vi "video.create_begin.vi"(8 "error in":errorcluster, 10 "name":string, 11 "Client in":refnum<class "Client.lvclass">) -> (0 "error out":errorcluster, 2 "VideoCreateStaging":refnum<class "VideoCreateStaging.lvclass">, 3 "Client out":refnum<class "Client.lvclass">)   [LabVIEW 2020, in "Client.lvclass"]
doc: "Creates a new empty video (metadata shell) with a name and optional description in Nominal and returns a handle to it."
uses:
  Client.lvclass
  Client.lvclass/Client.ctl
  client.lvlib
  VideoCreateStaging/VideoCreateStaging.lvclass
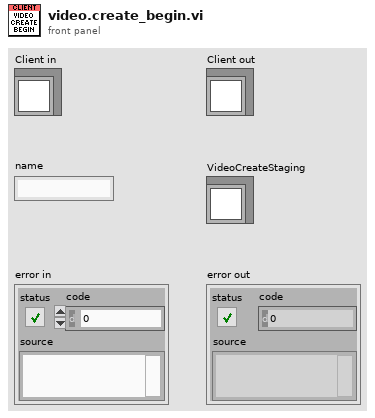
[diagram p1: front panel]
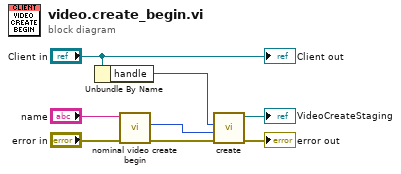
[diagram p0: block diagram]
diagram:
  n1 = Unbundle By Name("Client in") -> ("handle"=w3:i32)
  n2 = call "nominal video create begin.vi"("error in (no error)"="error in", "name"="name") -> ("error out"=w5:errorcluster, "out_staging out"=w2:i32)  [unwired: 7 in, 1 out]
  n3 = call "create.vi"("error in (no error)"=w5, "handle"=w2, "client"=w3) -> ("error out"=→"error out":errorcluster, "VideoCreateStaging out"=→"VideoCreateStaging":refnum<class "VideoCreateStaging.lvclass">)  [unwired: 7 in]
  "Client out" <- "Client in"
